vi "Initialize VIs Communication.vi"(8 "error in (no error)":errorcluster, 11 "Channel in":refnum<class "Channel.lvclass">) -> (0 "error out":errorcluster, 3 "Channel out":refnum<class "Channel.lvclass">)   [LabVIEW 2018, in "Channel.lvclass"]
doc: "Initialze the communcation with S4GUI"
uses:
  Channel.lvclass
  Channel.lvclass/Channel.ctl
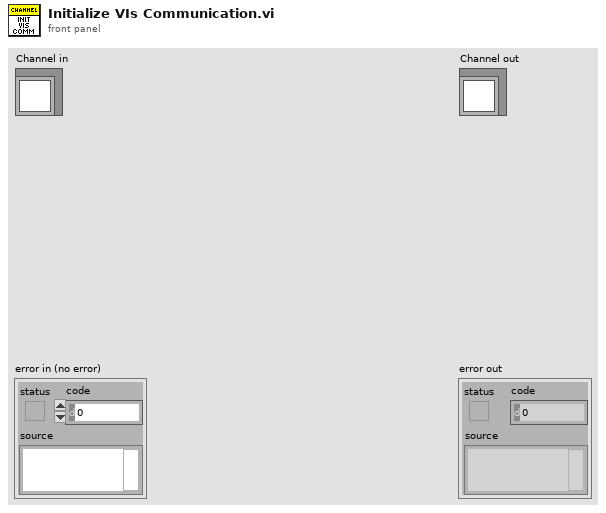
[diagram p1: front panel]
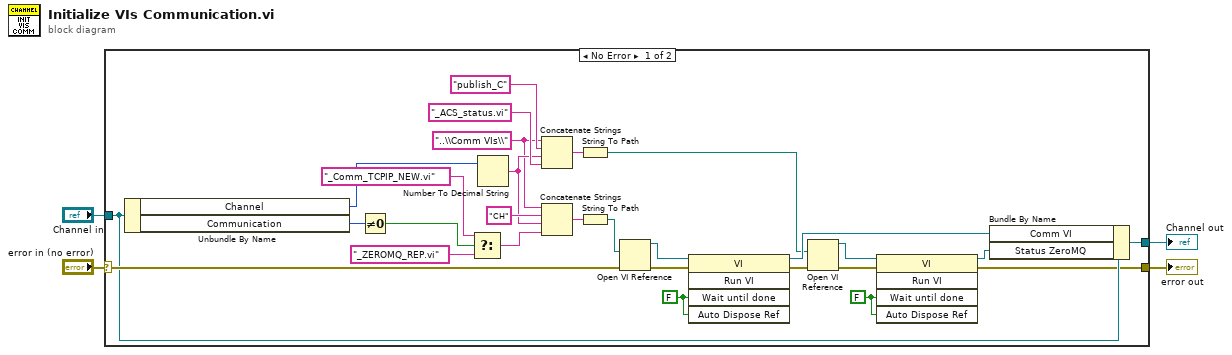
[diagram p0: block diagram]
diagram:
  n1 = case shown="No Error" "error in (no error)" {
    selector: "error in (no error)" -> [w27 w34]
    tunnel: [w14 w34] -> w3
    tunnel: [w15 w33] -> w1
    tunnel: "Channel in" -> [w23 w33]
    frame No Error {
      w5 = "..\\Comm VIs\\" ("name or relative path")
      w19 = FALSE ("Wait Until Done")
      w31 = FALSE ("Wait Until Done")
      n2 = Unbundle By Name(w23) -> ("Channel"=w10:u8, "Communication"=w6:u16)
      n3 = Not Equal To 0?(x=w6) -> (x != 0?=w7:bool)
      n4 = Select(t="_Comm_TCPIP_NEW.vi" ("name or relative path"), s=w7, f="_ZEROMQ_REP.vi" ("name or relative path")) -> (s? t:f=w25:string)
      n5 = Number To Decimal String(number=w10) -> (decimal integer string=w8:string)  [unwired: 1 in]
      n6 = Concatenate Strings(w5, "publish_C" ("name or relative path"), w8, "_ACS_status.vi" ("name or relative path")) -> (w11:string)
      n7 = Concatenate Strings(w5, "CH" ("name or relative path"), w8, w25) -> (w29:string)
      n8 = String To Path(string=w11) -> (path=w20:path)
      n9 = String To Path(string=w29) -> (path=w30:path)
      n10 = Open VI Reference(vi path=w30, error in (no error)=w27) -> (vi reference=w32:refnum<vi>, error out=w28:errorcluster)  [unwired: 4 in]
      n11 = invoke class="VI" method="Run VI"(reference=w32, error in=w28, "Wait until done"=w31, "Auto Dispose Ref"=w31) -> (reference out=w22:refnum<vi>, error out=w16:errorcluster)  [unwired: 1 in, 3 out]
      n12 = Open VI Reference(vi path=w20, error in (no error)=w16) -> (vi reference=w18:refnum<vi>, error out=w21:errorcluster)  [unwired: 4 in]
      n13 = invoke class="VI" method="Run VI"(reference=w18, error in=w21, "Wait until done"=w19, "Auto Dispose Ref"=w19) -> (reference out=w17:refnum<vi>, error out=w14:errorcluster)  [unwired: 1 in, 3 out]
      n14 = Bundle By Name(cluster=w23, "Comm VI"=w22, "Status ZeroMQ"=w17) -> (w15:refnum<class "Channel.lvclass">)
    }
    frame Error {
    }
  }
  "error out" <- w3
  "Channel out" <- w1
